vi "controlled_clock.vi"() -> ()   [LabVIEW 2017]
panel:
  in  "seconds":dbl(knob) scale=0.0..11.0
  in  "minutes":dbl(knob) scale=0.0..11.0
  in  "hours":dbl(knob) scale=0.0..11.0
  out "Gauge":cluster{dbl, dbl, dbl}(knob)={0.0, 0.0, 10.283060822363773} scale=0.0..11.0
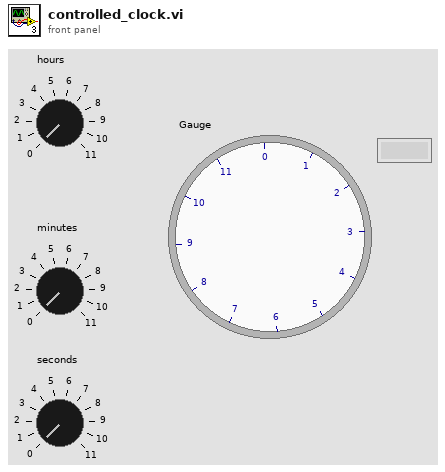
[diagram p1: front panel]
types:
  T1 = cluster{"hours":dbl, "minutes":dbl, "seconds":dbl}
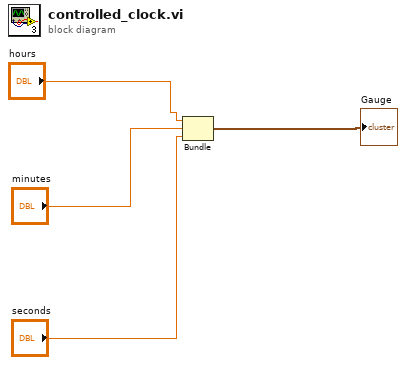
[diagram p0: block diagram]
diagram:
  n1 = Bundle("hours"="hours", "minutes"="minutes", "seconds"="seconds") -> (→"Gauge":T1)  [unwired: 1 in]
